vi "GUI_HTU_148Pico.vi"() -> ()   [LabVIEW 2013]
uses:
  Shared/GUI_Template/GUI_master/tcp_new_data_event.ctl
  Shared/GUI_Template/GUI_master/tcp new data cluster.ctl
panel:
  in  "Position.Axis 311::1":dbl caption="Expander In 1 Y" min=-999999.0 max=999999.0
  in  "Position.Axis 243::1":dbl caption="Expander In 1 X" min=-999999.0 max=999999.0
  in  "Position.Axis 223::1":dbl caption="Gaia3 North Y" min=-999999.0 max=999999.0
  in  "Position.Axis 222::1":dbl caption="Gaia3 North X" min=-999999.0 max=999999.0
  in  "Position.Axis 322::1":dbl caption="Gaia2 North Y" min=-999999.0 max=999999.0
  in  "Position.Axis 321::1":dbl caption="Gaia2 North X" min=-999999.0 max=999999.0
  in  "Position.Axis 242::1":dbl caption="Gaia4 North Y" min=-999999.0 max=999999.0
  in  "Position.Axis 241::1":dbl caption="Gaia4 North X" min=-999999.0 max=999999.0
  in  "Position.Axis 132::1":dbl caption="Gaia2 South Y" min=-999999.0 max=999999.0
  in  "Position.Axis 323::1":dbl caption="Gaia2 South X" min=-999999.0 max=999999.0
  in  "Position.Axis 143::1":dbl caption="Gaia4 South Y" min=-999999.0 max=999999.0
  in  "Position.Axis 142::1":dbl caption="Gaia4 South X" min=-999999.0 max=999999.0
  in  "Position.Axis 141::1":dbl caption="Gaia3 South Y" min=-999999.0 max=999999.0
  in  "Position.Axis 133::1":dbl caption="Gaia3 South X" min=-999999.0 max=999999.0
  in  "Position.Axis 313::1":dbl caption="Amp4 Out Y" min=-999999.0 max=999999.0
  in  "Position.Axis 221::1":dbl caption="Amp4 Out X" min=-999999.0 max=999999.0
  in  "Position.Axis 213::1":dbl caption="Amp2 In Y" min=-999999.0 max=999999.0
  in  "Position.Axis 211::1":dbl caption="Amp2 In X" min=-999999.0 max=999999.0
  in  "Position.Axis 123::1":dbl caption="Amp4 In Y" min=-999999.0 max=999999.0
  in  "Position.Axis 131::1":dbl caption="Amp4 In X" min=-999999.0 max=999999.0
  in  "Position.Axis 121::1":dbl caption="Amp3 In Y" min=-999999.0 max=999999.0
  in  "Position.Axis 113::1":dbl caption="Amp3 In X" min=-999999.0 max=999999.0
  in  "Position.Axis 112::1":dbl caption="Amp2 Out Y" min=-999999.0 max=999999.0
  in  "Position.Axis 111::1":dbl caption="Amp2 Out X" min=-999999.0 max=999999.0
  out "tcp data event":T1
  out "error IO 2":errorcluster
  in  "GUIdevice 1":string="U_148_PicoServer"
  in  "?":bool
  # "Gaia motors"
  # "Amplifier motors"
  # "South"
  # "North"
  # "Expander In motors"
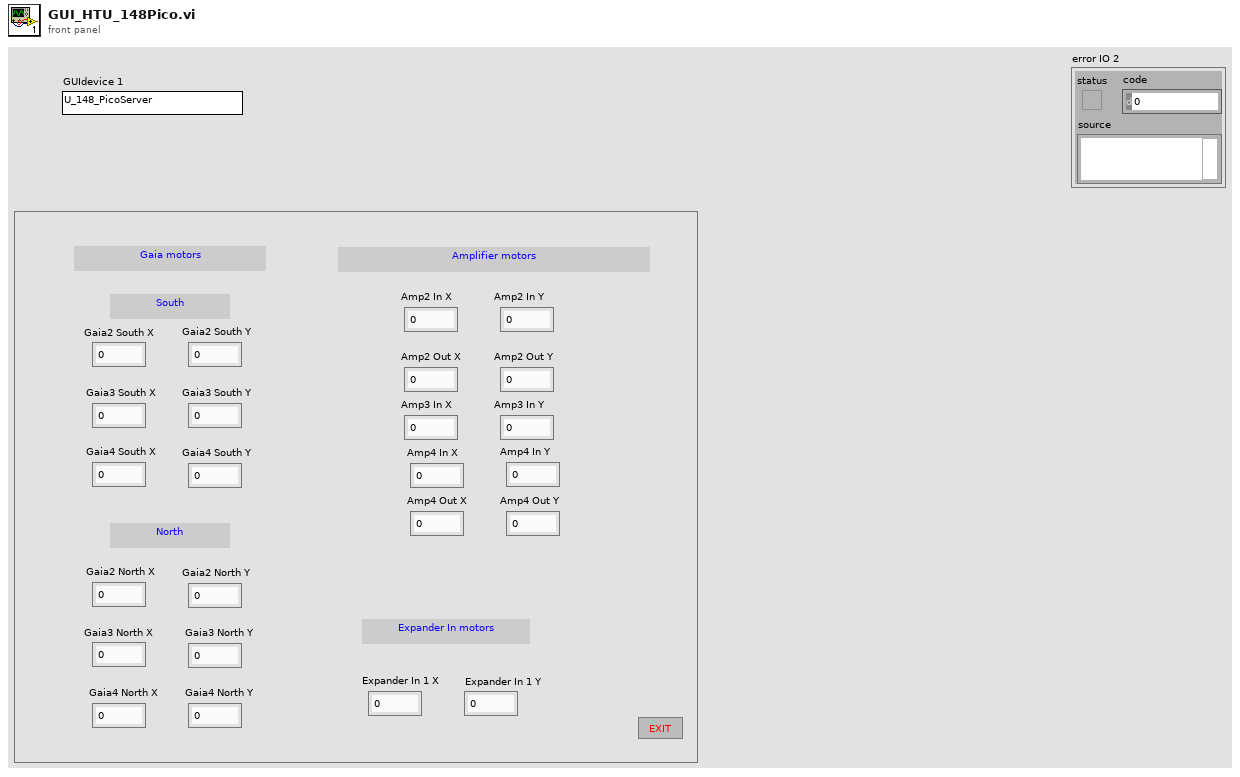
[diagram p1: front panel]
types:
  T1 = typedef "tcp_new_data_event.ctl" = refnum<user-event>
  T2 = typedef "tcp new data cluster.ctl" = cluster{"EventEnum":enum16{"new data", "connection status update"}, "Device name":string}
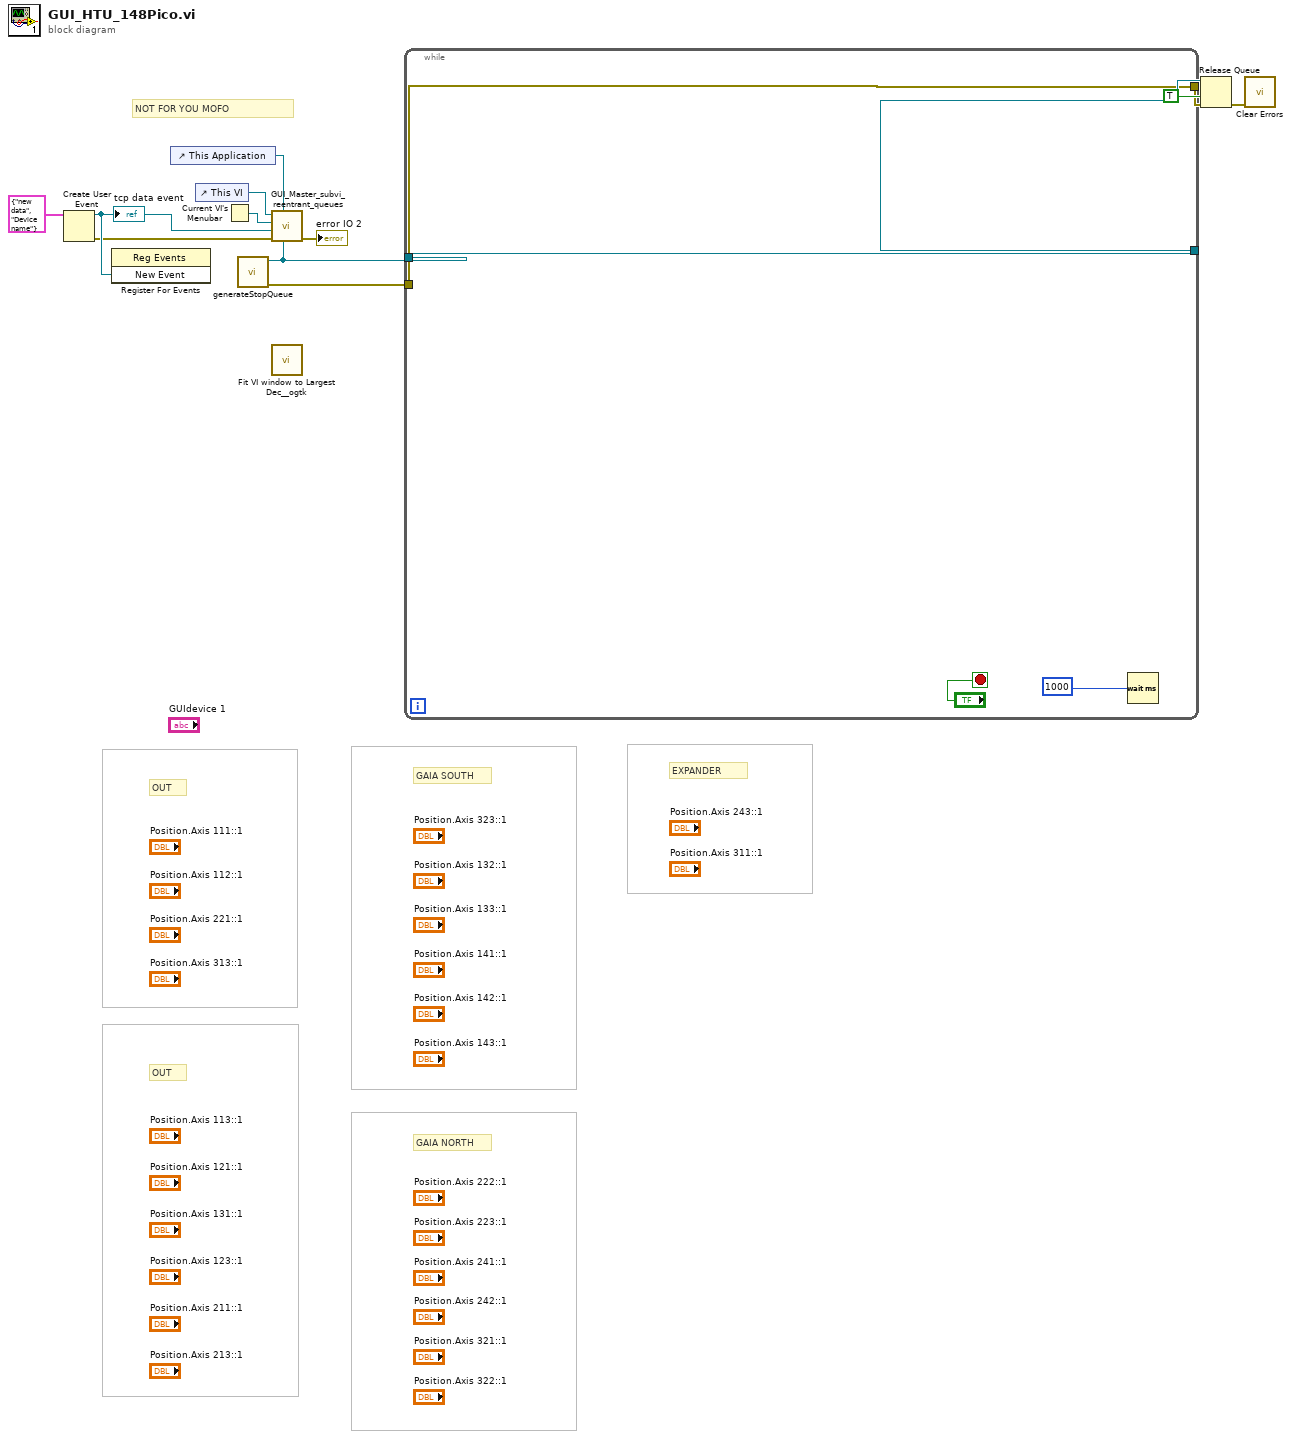
[diagram p0: block diagram]
diagram:
  # "OUT"
  # "OUT"
  # "EXPANDER"
  # "GAIA NORTH"
  # "GAIA SOUTH"
  # "NOT FOR YOU MOFO"
  n1 = Create User Event(user event datatype=T2 {"EventEnum"=enum."new data", "Device name"="Device name"} ("New Event")) -> (user event=w8:refnum<user-event>, error out=w7:errorcluster)  [unwired: 1 in]
  "tcp data event" <- w8
  n2 = register-events(w8) -> ()  [unwired: 2 in, 2 out]
  n3 = control-ref of="This Application"() -> (w9:refnum<vi>)
  n4 = control-ref of="This VI"() -> (w4:refnum<vi>)
  n5 = Current VI's Menubar() -> (w5:refnum<k9>)
  n6 = call "generateStopQueue.vi"() -> ("error out"=w2:errorcluster, "STOP Queue out"=w1:refnum<queue>)  [unwired: 10 in]
  n7 = call "GUI_Master_subvi_reentrant_queues.vi"("STOP Queue in"=w1, "This Application"=w9, "error in (no error)"=w7, "tcp data event"=w8, "Caller menu reference"=w5, "Caller VI ref"=w4) -> ("error out"=→"error IO 2":errorcluster)  [unwired: 5 in]
  n8 = call <userlib>:"Fit VI window to Largest Dec__ogtk.vi"() -> ()  [unwired: 6 in, 2 out]
  n9 = while {
    tunnel: [w16] -> w11
    tunnel: w2 -> [w16]
    tunnel: w1 -> [w15]
    tunnel: [w15] -> w10
    stop <- "?" stop-if-true
    n10 = Wait (ms)(milliseconds to wait=u32 1000) -> ()  [unwired: 1 out]
  }
  n11 = Release Queue(queue=w10, force destroy? (F)=TRUE, error in (no error)=w11) -> (error out=w13:errorcluster)  [unwired: 2 out]
  n12 = call <vilib>:"Clear Errors.vi"("error in (no error)"=w13) -> ()  [unwired: 6 in, 1 out]
